vi "Scale Intensity Graph.vi"(8 "error in (no error)":errorcluster, 11 "IntensityGraph in":refnum<vi>) -> (0 "error out":errorcluster, 2 "marker vals":cluster{dbl, "Color Box":u32}[](array[cluster]), 3 "IntensityGraph out":refnum<vi>)   [LabVIEW 2014]
doc: "Scales the graph and sets the marker vals accordingly"
uses:
  MSC Image_class/controls/Image Type.ctl
  MSC Image_class/MSC Image.lvclass
panel:
  in  "Type":T1 items=["Grayscale U8"=0, "Grayscale U16"=2, "Grayscale Single"=5, "Grayscale Double"=6, "RGB U8"=16]
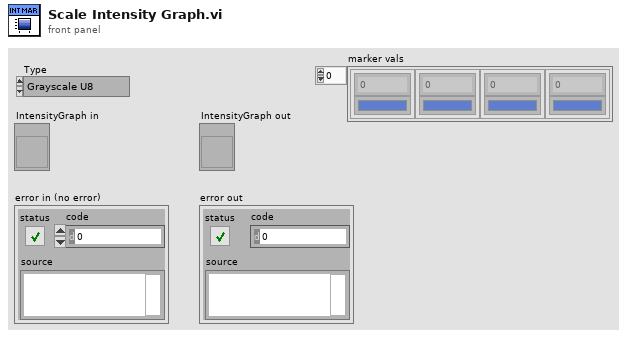
[diagram p1: front panel]
types:
  T1 = typedef "MSC Image.lvclass/Image Type.ctl" = i32
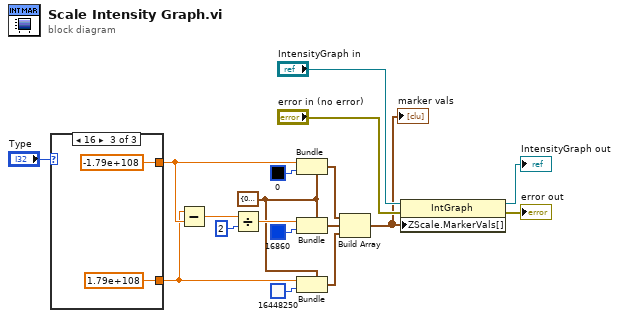
[diagram p0: block diagram]
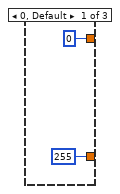
[diagram p2: hidden frame]
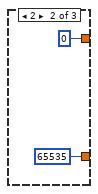
[diagram p3: hidden frame]
diagram:
  w2 = cluster{dbl, u32} {0.0, 0}
  n1 = case shown="16" "Type" {
    tunnel: [0 0 -1.79e+108] -> w11
    tunnel: [255 65535 1.79e+108] -> w7
    frame 0, Default {
    }
    frame 2 {
    }
    frame 16 {
    }
  }
  n2 = Subtract(x=w7, y=w11) -> (x-y=w13:dbl)
  n3 = Divide(x=w13, y=2) -> (x/y=w9:dbl)
  n4 = Bundle(cluster=w2, w11, u32 0) -> (w5:cluster{dbl, u32})
  n5 = Bundle(cluster=w2, w9, u32 16860) -> (w4:cluster{dbl, u32})
  n6 = Bundle(cluster=w2, w7, u32 16448250) -> (w3:cluster{dbl, u32})
  n7 = Build Array(w5, w4, w3) -> (w1:cluster{dbl, u32}[])
  "marker vals" <- w1
  n8 = property on="Property Node" class="IntGraph"(reference="IntensityGraph in", error in="error in (no error)", "ZScale.MarkerVals[]"=w1) -> (reference out=→"IntensityGraph out":refnum<vi>, error out=→"error out":errorcluster)
